vi "Create.vi"(8 "error in (no error)":errorcluster caption="错误输入（无错误）", 11 "FileSystem 输入":refnum<class "FileSystem.lvclass"> caption="DNL_LabVIEW Object in") -> (0 "error out":errorcluster caption="错误输出", 3 "FileSystem 输出":refnum<class "FileSystem.lvclass"> caption="DNL_LabVIEW Object out")   [LabVIEW 2012, in "FileSystem.lvclass"]
uses:
  FileSystem.lvclass
  FileSystem.lvclass/FileSystem.ctl
  Microsoft.VisualBasic
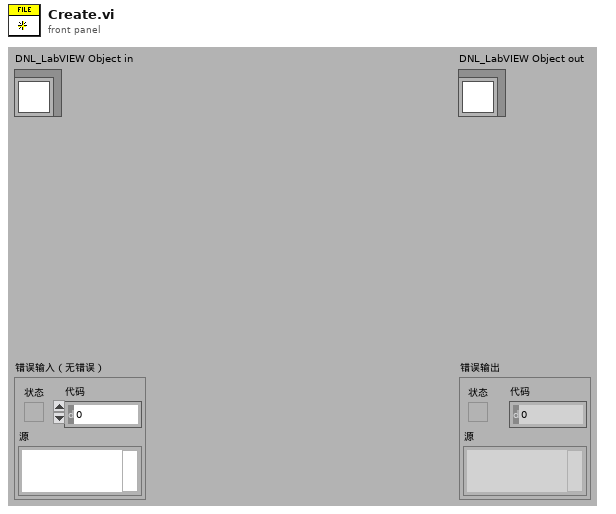
[diagram p1: front panel]
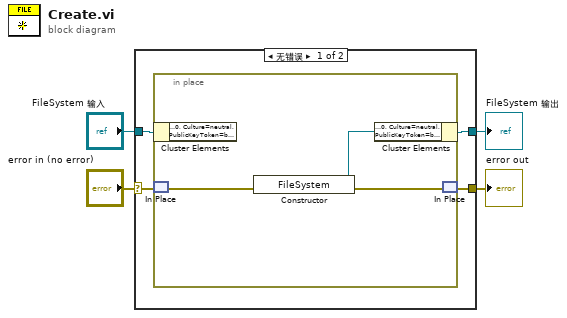
[diagram p0: block diagram]
diagram:
  n1 = case shown="无错误" "error in (no error)" {
    selector: "error in (no error)" -> [w6 w13]
    tunnel: [w5 w13] -> w3
    tunnel: [w7 w12] -> w1
    tunnel: "FileSystem 输入" -> [w8 w12]
    frame No Error {
      n2 = in-place {
        n3 = in-place-cluster #1(w8) -> ()  [unwired: 1 out]
        n4 = in-place-match #2(w6) -> (w10:errorcluster)
        n5 = constructor class="FileSystem"(error in=w10) -> (reference out=w11:refnum<k24>, error out=w9:errorcluster)  [unwired: 2 in, 1 out]
        n6 = in-place-cluster #1("FileSystem"=w11) -> (w7:refnum<class "FileSystem.lvclass">)
        n7 = in-place-match #2(w9) -> (w5:errorcluster)
      }
    }
    frame Error {
    }
  }
  "error out" <- w3
  "FileSystem 输出" <- w1
